vi "Get all Targets.vi"(7 "App instance":refnum<vi>, 8 "error in":errorcluster, 11 "Project Selection":string) -> (0 "error out":errorcluster, 3 "Targets":string[](array[string]))   [LabVIEW 2019, in "Panther Dashboard.lvlib"]
uses:
  Panther Dashboard.lvlib
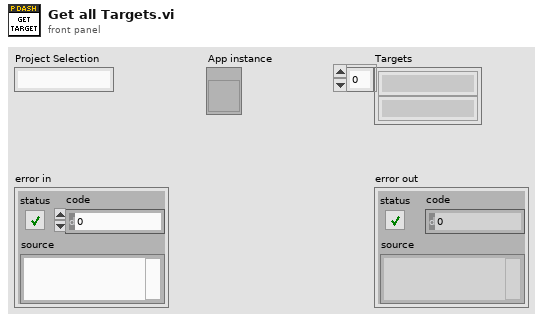
[diagram p1: front panel]
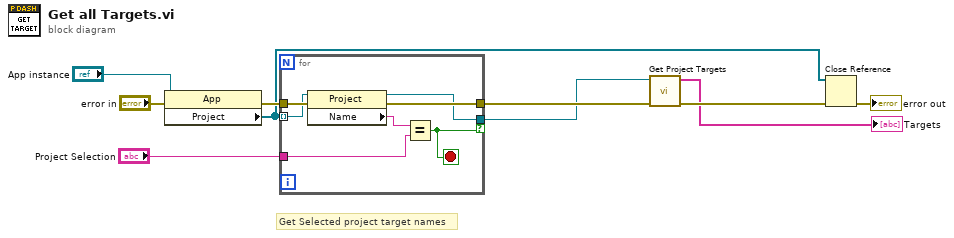
[diagram p0: block diagram]
diagram:
  # "Get Selected project target names"
  n1 = property class="App"(reference="App instance", error in="error in") -> (error out=w9:errorcluster, "Project"=w2:refnum<vi>[])  [unwired: 1 out]
  n2 = for {
    tunnel: w2 -> [w15] mode=indexing
    tunnel: [w12] -> w5 if=w11
    tunnel: "Project Selection" -> [w13]
    tunnel: w9 -> [w17]
    tunnel: [w16] -> w8
    stop <- w11 stop-if-true
    n3 = property class="Project"(reference=w15, error in=w17) -> (reference out=w12:refnum<vi>, error out=w16:errorcluster, "Name"=w14:string)
    n4 = Equal?(x=w14, y=w13) -> (x = y?=w11:bool)
  }
  n5 = call "Get Project Targets.vi"("error in"=w8, "Project in"=w5) -> ("error out"=w6:errorcluster, "Targets"=→"Targets":string[])  [unwired: 8 in]
  n6 = Close Reference(reference=w2, error in (no error)=w6) -> (error out=→"error out":errorcluster)
